vi "client.vi"() -> (0 "error":bool, 3 "value":i32[][](array[numeric]))   [LabVIEW 2022 SP3]
doc: "This VI implements a client for the TCP Named Service - Server.vi. It connects to a service by specifying the server address and the name of the service. The client receives the string sent by the server, displays the string and closes the connection."
panel:
  out "valueString":string
  out "Message from Server":string
  # "從網路上(須找到名為2OtheFlooR234的server)接收資料(為一字串)，並轉換為8*8的陣列"
  # "Overview: Demonstrates the use of the TCP functions to connect to a TCP server VI via named service and receive data.\nInstructions:\n1. Ensure TCP Named Service - Server.vi is already running.\n2. Run the VI."
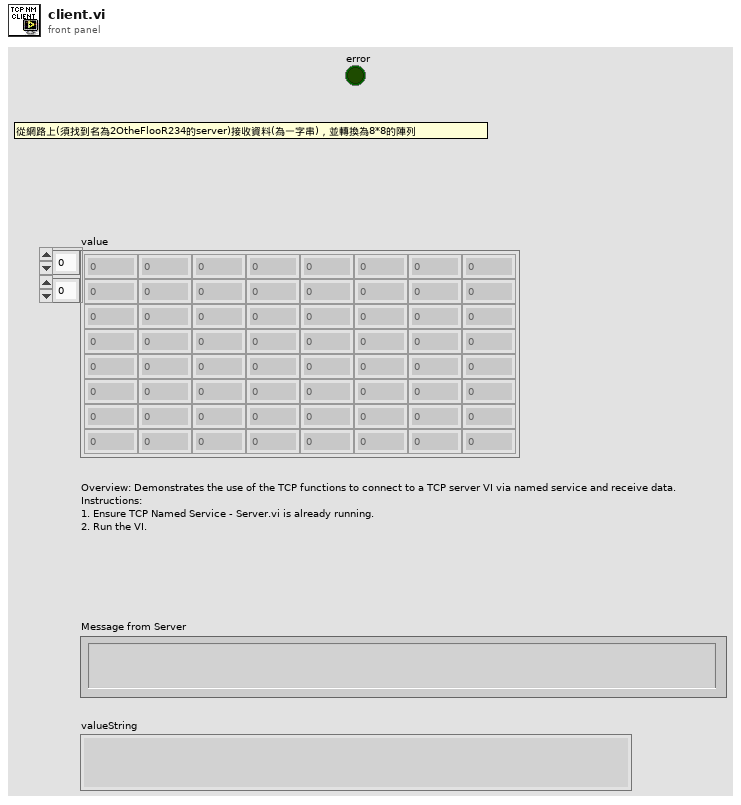
[diagram p1: front panel]
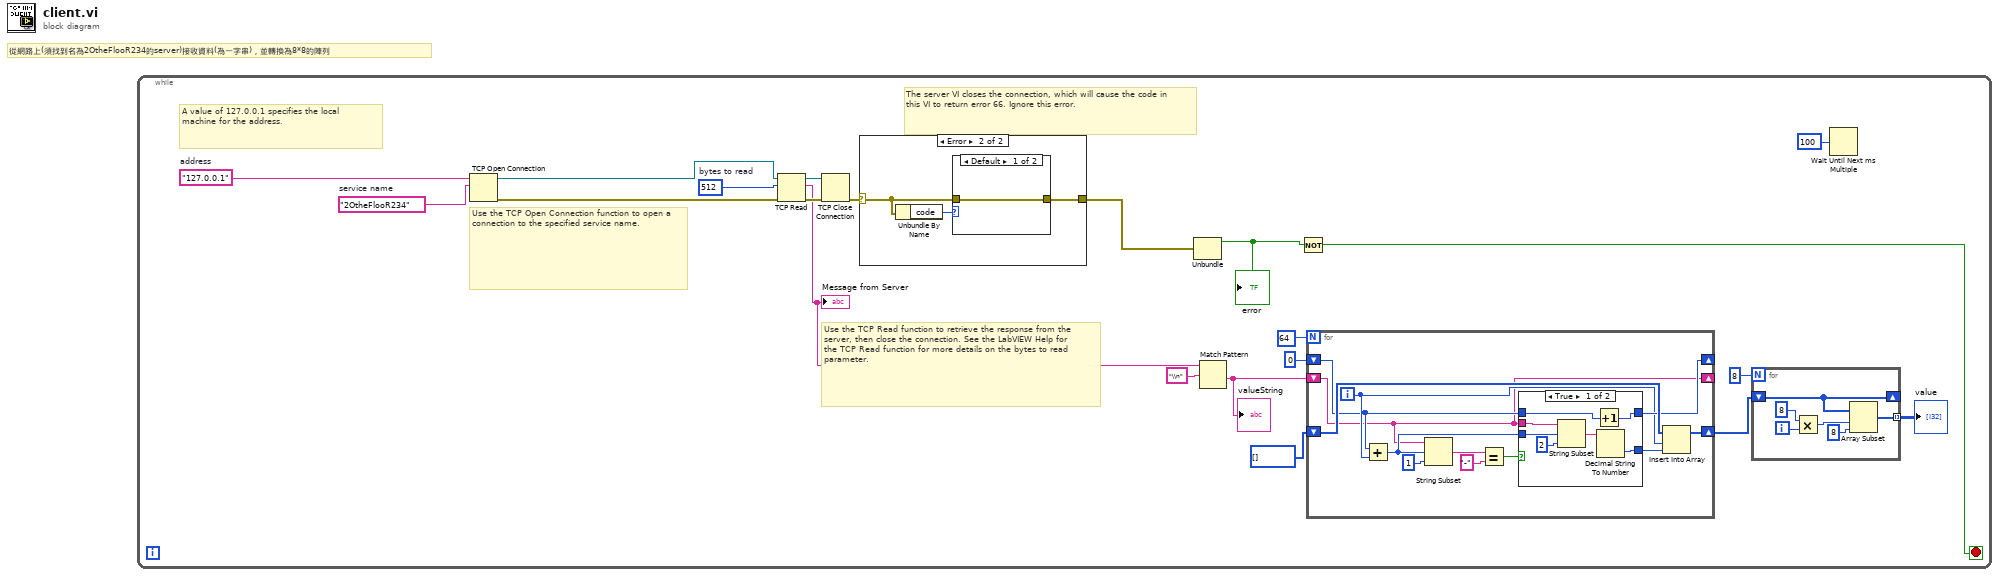
[diagram p0: block diagram]
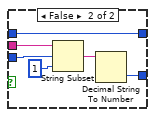
[diagram p2: hidden frame]
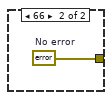
[diagram p4: hidden frame]
diagram:
  # "從網路上(須找到名為2OtheFlooR234的server)接收資料(為一字串)，並轉換為8*8的陣列"
  n1 = while {
    stop <- w2 stop-if-true
    w15 = 512  # bytes to read
    w16 = "2OtheFlooR234"  # service name
    w17 = "127.0.0.1"  # address
    # "The server VI closes the connection, which will cause the code in this VI to return error 66. Ignore this error."
    # "A value of 127.0.0.1 specifies the local machine for the address."
    # "Use the TCP Open Connection function to open a connection to the specified service name."
    # "Use the TCP Read function to retrieve the response from the server, then close the connection. See the LabVIEW Help for the TCP Read function for more details on the bytes to read parameter."
    n2 = TCP Open Connection(address=w17, remote port or service name=w16) -> (connection ID=w20:refnum<k5>, error out=w21:errorcluster)  [unwired: 3 in]
    n3 = TCP Read(connection ID=w20, bytes to read=w15, error in (no error)=w21) -> (connection ID out=w19:refnum<k5>, data out=w12:string, error out=w18:errorcluster)  [unwired: 2 in]
    "Message from Server" <- w12
    n4 = TCP Close Connection(connection ID=w19, error in (no error)=w18) -> (error out=w14:errorcluster)  [unwired: 1 in, 1 out]
    n5 = case shown="Error" w14 {
      selector: w14 -> [w53 w55]
      tunnel: [w53 w54] -> w4
      frame No Error {
      }
      frame Error {
        n6 = Unbundle By Name(w55) -> ("code"=w56:i32)
        n7 = case shown="Default" w56 {
          tunnel: w55 -> [w57 _]
          tunnel: [w57 w58] -> w54
          frame Default {
          }
          frame 66 {
            w58 = errorcluster {"status"=FALSE, "code"=0, "source"=""}  # No error
          }
        }
      }
    }
    n8 = Unbundle(w4) -> ("status"=w3:bool)  [unwired: 2 out]
    "error" <- w3
    n9 = Match Pattern(string=w12, regular expression="\\n") -> (after substring=w10:string)  [unwired: 1 in, 3 out]
    "valueString" <- w10
    n10 = Not(x=w3) -> (.not. x?=w2:bool)
    n11 = for {
      N: 64 -> [_]
      shift-right: [w28] -> _
      shift-left: w10 -> [w28]
      shift-right: [w38] -> w6
      shift-left: i32[] [] -> [w39]
      shift-right: [w32] -> _
      shift-left: 0 -> [w30]
      i -> [w31]
      n12 = Add(x=w30, y=w31) -> (x+y=w29:i32)
      n13 = String Subset(string=w28, offset (0)=w29, length (rest)=1 ("length (rest)")) -> (substring=w36:string)
      n14 = Equal?(x=w36, y="-") -> (x = y?=w34:bool)
      n15 = case shown="True" w34 {
        tunnel: [w46 w52] -> w33
        tunnel: w28 -> [w45 w51]
        tunnel: w30 -> [w42 w48]
        tunnel: [w41 w48] -> w32
        tunnel: w29 -> [w40 w47]
        frame True {
          n16 = String Subset(string=w45, offset (0)=w40, length (rest)=2 ("length (rest)")) -> (substring=w43:string)
          n17 = Increment(x=w42) -> (x+1=w41:i32)
          n18 = Decimal String To Number(string=w43) -> (number=w46:i32)  [unwired: 2 in, 1 out]
        }
        frame False {
          n19 = String Subset(string=w51, offset (0)=w47, length (rest)=1 ("length (rest)")) -> (substring=w49:string)
          n20 = Decimal String To Number(string=w49) -> (number=w52:i32)  [unwired: 2 in, 1 out]
        }
      }
      n21 = Insert Into Array(array=w39, index=w31, new element=w33) -> (w38:i32[])
    }
    n22 = for {
      N: 8 -> [_]
      shift-right: [w27] -> _
      shift-left: w6 -> [w27]
      tunnel: [w22] -> w5 mode=indexing
      i -> [w25]
      n23 = Multiply(x=8, y=w25) -> (x*y=w24:i32)
      n24 = Array Subset(array=w27, index=w24, length=8) -> (w22:i32[])
    }
    "value" <- w5
    n25 = Wait Until Next ms Multiple(millisecond multiple=u32 100) -> ()  [unwired: 1 out]
  }
